vi "SubPanel_InsertVI.vi"(7 "SubPanVI_Names":string[](array[string]), 8 "error in (no error)":errorcluster, 9 "SubPanRefs":refnum<vi>[](array[refnum]), 10 "InsertVI_Name":string, 11 "SubPanel in":refnum<vi>) -> (0 "error out":errorcluster, 3 "InsertedVI":refnum<vi>)   [LabVIEW 2014, in "SubPanelModule.lvlib"]
uses:
  SubPanelModule.lvlib
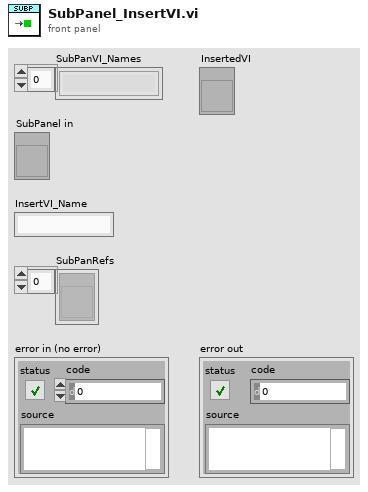
[diagram p1: front panel]
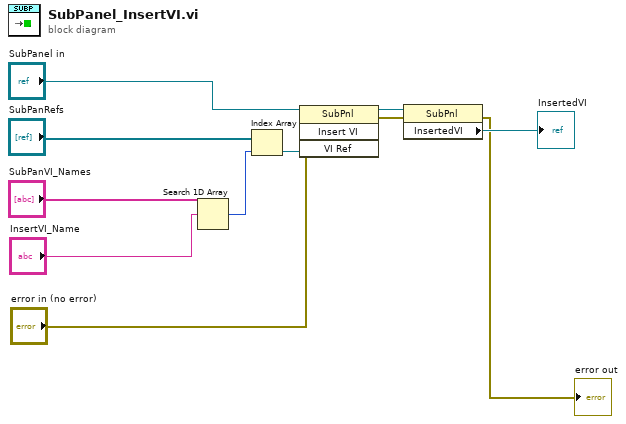
[diagram p0: block diagram]
diagram:
  n1 = Search 1D Array(1D array="SubPanVI_Names", element="InsertVI_Name") -> (index of element=w10:i32)  [unwired: 1 in]
  n2 = Index Array(array="SubPanRefs", index=w10) -> (element=w11:refnum<vi>)
  n3 = invoke class="SubPnl" method="Insert VI"(reference="SubPanel in", error in="error in (no error)", "VI Ref"=w11) -> (reference out=w4:refnum<vi>, error out=w3:errorcluster)  [unwired: 1 in, 2 out]
  n4 = property class="SubPnl"(reference=w4, error in=w3) -> (error out=→"error out":errorcluster, "InsertedVI"=→"InsertedVI":refnum<vi>)  [unwired: 1 out]
